vi "open_magazine.vi"(8 "error in (no error)":errorcluster) -> (0 "error out":errorcluster)   [LabVIEW 2020]
uses:
  <vilib>/Rock Robotics/WPI/ThirdParty/Phoenix-LabVIEW/Motor Controller/Controls/CTRE_Phoenix_MotorControl_NeutralMode.ctl
  Status Frame Stuff/Talon Status Config Array.ctl
  Status Frame Stuff/Talon Status Frame Setting.ctl
  <vilib>/Rock Robotics/WPI/ThirdParty/Phoenix-LabVIEW/Motor Controller/Controls/CTRE_Phoenix_MotorControl_StatusFrameEnhanced.ctl
  Status Frame Stuff/STATUS_Period.ctl
  <vilib>/Rock Robotics/SystemInterfaces/DIO/FPGA_DIOChannel.ctl
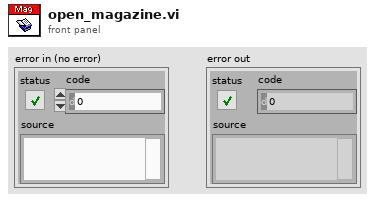
[diagram p1: front panel]
types:
  T1 = typedef "FPGA_DIOChannel.ctl" = enum8{"DIO 0", "DIO 1", "DIO 2", "DIO 3", "DIO 4", "DIO 5", "DIO 6", "DIO 7", "DIO 8", "DIO 9", "DIO MXP 0", "DIO MXP 1", "DIO MXP 2", "DIO MXP 3", "DIO MXP 4", "DIO MXP 5", "DIO MXP 6", "DIO MXP 7", "DIO MXP 8", "DIO MXP 9", "DIO MXP 10", "DIO MXP 11", "DIO MXP 12", "DIO MXP 13", "DIO MXP 14", "DIO MXP 15", "SPI Port CS1", "SPI Port CS2", "SPI Port CS3", "SPI Port MISO", "SPI Port MOSI", "Invalid"}
  T2 = typedef "Talon Status Config Array.ctl" = T3[]
  T3 = typedef "Talon Status Frame Setting.ctl" = cluster{"Status Frame Enum":T4, "STATUS_Period":T5}
  T4 = typedef "CTRE_Phoenix_MotorControl_StatusFrameEnhanced.ctl" = u16
  T5 = typedef "STATUS_Period.ctl" = i32
  T6 = typedef "CTRE_Phoenix_MotorControl_NeutralMode.ctl" = enum8{"EEPROMSetting", "Override to Coast", "Override to Brake"}
  T7 = typedef "WPI_MotorControlDeviceRef.ctl" = cluster{"DeviceStatus":errorcluster, "Type":T8, "PWM":cluster{"PWM Channel":T9, "DeadBand":T10}, "CAN":cluster{"Device Number":u8, "SetOutput VI Ref":variant, "GetOutput VI Ref":variant, "Enable VI Ref":variant, "Disable VI Ref":variant, "Data":variant}, "Invert":bool, "DIO PWM":cluster{"PWM \"Enable\" Channel":T9, "DIOChannel":T1, "PWM Rate":dbl}}
  T8 = typedef "WPI_MotorControlType.ctl" = enum16{"PWM", "CAN", "DIO PWM"}
  T9 = typedef "FPGA_DIOPWMChannel.ctl" = enum8{"PWM 0", "PWM 1", "PWM 2", "PWM 3", "PWM 4", "PWM 5", "PWM 6", "PWM 7", "PWM 8", "PWM 9", "PWM MXP 0", "PWM MXP 1", "PWM MXP 2", "PWM MXP 3", "PWM MXP 4", "PWM MXP 5", "PWM MXP 6", "PWM MXP 7", "PWM MXP 8", "PWM MXP 9", "Invalid"}
  T10 = typedef "WPI_PWMDeadband.ctl" = cluster{"Name":string, "maxPositivePwm":i32, "minPositivePwm":i32, "centerPwm":i32, "maxNegativePwm":i32, "minNegativePwm":i32, "angularRange":u16}
  T11 = typedef "WPI_DigitalInputDevRef.ctl" = cluster{"DevStatus":errorcluster, "DIO Channel":T1}
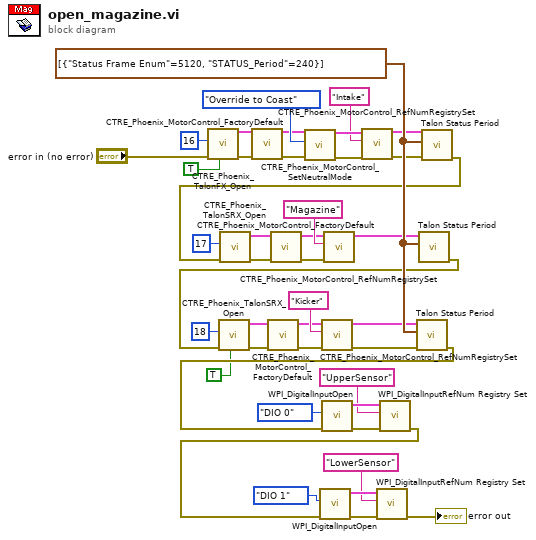
[diagram p0: block diagram]
diagram:
  w42 = T2 [{"Status Frame Enum"=5120, "STATUS_Period"=240}] ("Drive Status Config")
  n1 = call <vilib>:"CTRE_Phoenix_TalonFX_Open.vi"("Invert"=TRUE, "error in"="error in (no error)", "Device Number"=u8 16) -> ("error out"=w13:errorcluster, "PhoenixMotorControlDevRef"=w14:T7)  [unwired: 7 in]
  n2 = call <vilib>:"CTRE_Phoenix_MotorControl_FactoryDefault.vi"("error in"=w13, "PhoenixMotorControlDevRef"=w14) -> ("error out"=w18:errorcluster, "PhoenixMotorControlDevRef"=w17:T7)  [unwired: 8 in]
  n3 = call <vilib>:"CTRE_Phoenix_MotorControl_SetNeutralMode.vi"("error in (no error)"=w18, "Motor Control Neutral Mode"=CTRE_Phoenix_MotorControl_NeutralMode."Override to Coast", "PhoenixMotorControlDevRef"=w17) -> ("error out"=w20:errorcluster, "PhoenixMotorControlDevRef"=w19:T7)  [unwired: 7 in]
  n4 = call <vilib>:"CTRE_Phoenix_MotorControl_RefNumRegistrySet.vi"("error in (no error)"=w20, "refnum name"="Intake", "PhoenixMotorControlDevRef"=w19) -> ("error out"=w36:errorcluster, "PhoenixMotorControlDevRef"=w35:T7)  [unwired: 7 in]
  n5 = call "Talon Status Period.vi"("error in (no error)"=w36, "Status Config Array"=w42, "PhoenixMotorControlDevRef"=w35) -> ("error out"=w37:errorcluster)  [unwired: 7 in, 1 out]
  n6 = call <vilib>:"CTRE_Phoenix_TalonSRX_Open.vi"("error in"=w37, "Device Number"=u8 17) -> ("error out"=w22:errorcluster, "PhoenixMotorControlDevRef"=w23:T7)  [unwired: 8 in]
  n7 = call <vilib>:"CTRE_Phoenix_MotorControl_FactoryDefault.vi"("error in"=w22, "PhoenixMotorControlDevRef"=w23) -> ("error out"=w26:errorcluster, "PhoenixMotorControlDevRef"=w27:T7)  [unwired: 8 in]
  n8 = call <vilib>:"CTRE_Phoenix_MotorControl_RefNumRegistrySet.vi"("error in (no error)"=w26, "refnum name"="Magazine", "PhoenixMotorControlDevRef"=w27) -> ("PhoenixMotorControlDevRef"=w38:T7)  [unwired: 7 in, 1 out]
  n9 = call "Talon Status Period.vi"("Status Config Array"=w42, "PhoenixMotorControlDevRef"=w38) -> ("error out"=w39:errorcluster)  [unwired: 8 in, 1 out]
  n10 = call <vilib>:"CTRE_Phoenix_TalonSRX_Open.vi"("Invert"=TRUE, "error in"=w39, "Device Number"=u8 18) -> ("error out"=w24:errorcluster, "PhoenixMotorControlDevRef"=w25:T7)  [unwired: 7 in]
  n11 = call <vilib>:"CTRE_Phoenix_MotorControl_FactoryDefault.vi"("error in"=w24, "PhoenixMotorControlDevRef"=w25) -> ("error out"=w28:errorcluster, "PhoenixMotorControlDevRef"=w29:T7)  [unwired: 8 in]
  n12 = call <vilib>:"CTRE_Phoenix_MotorControl_RefNumRegistrySet.vi"("error in (no error)"=w28, "refnum name"="Kicker", "PhoenixMotorControlDevRef"=w29) -> ("error out"=w41:errorcluster, "PhoenixMotorControlDevRef"=w40:T7)  [unwired: 7 in]
  n13 = call "Talon Status Period.vi"("error in (no error)"=w41, "Status Config Array"=w42, "PhoenixMotorControlDevRef"=w40) -> ("error out"=w4:errorcluster)  [unwired: 7 in, 1 out]
  n14 = call <vilib>:"WPI_DigitalInputOpen.vi"("error in (no error)"=w4, "DIO Channel"=FPGA_DIOChannel."DIO 0") -> ("error out"=w9:errorcluster, "DigitalInputDevRef"=w10:T11)  [unwired: 8 in]
  n15 = call <vilib>:"WPI_DigitalInputRefNum Registry Set.vi"("error in (no error)"=w9, "refnum name"="UpperSensor", "DigitalInputDevRef"=w10) -> ("error out"=w3:errorcluster)  [unwired: 7 in, 1 out]
  n16 = call <vilib>:"WPI_DigitalInputOpen.vi"("error in (no error)"=w3, "DIO Channel"=FPGA_DIOChannel."DIO 1") -> ("error out"=w11:errorcluster, "DigitalInputDevRef"=w12:T11)  [unwired: 8 in]
  n17 = call <vilib>:"WPI_DigitalInputRefNum Registry Set.vi"("error in (no error)"=w11, "refnum name"="LowerSensor", "DigitalInputDevRef"=w12) -> ("error out"=→"error out":errorcluster)  [unwired: 7 in, 1 out]
